vi "HDF5_Write_Filter_Record.vi"(0 "Filter_Refs":T2 {"Filter_Group_ref" format="%.0x"; "TimeStamp_dset" format="%.0x"; "Filter_dset" format="%.0x"}, 5 "Config.FP_User.1.FilterEnab":T1=enum."Step 1", 11 "error in":errorcluster) -> (15 "error out":errorcluster)   [LabVIEW 2018]
doc: "Write a single Noise<x> record with timestamp:\nNoise1\n NoiseInfo - cluster with Timestamp and other metadata for this record\n SummdSpectrum - 1024 element Double array (waveform)"
uses:
  HDF5_Filter_refs.ctl
  <vilib>/addons/h5labview2/base/hid_t.ctl
  Controls/RadioButtons/FilterEnableRadio.ctl
  <vilib>/addons/h5labview2/base/lib_path.vi
  <vilib>/addons/h5labview2/base/H5Equery.vi
  <vilib>/addons/h5labview2/dataset/H5Dwrite.llb/H5Dwrite.xnode
  <vilib>/addons/h5labview2/dataset/H5D.lvlib
  <vilib>/addons/h5labview2/space/H5S.lvlib
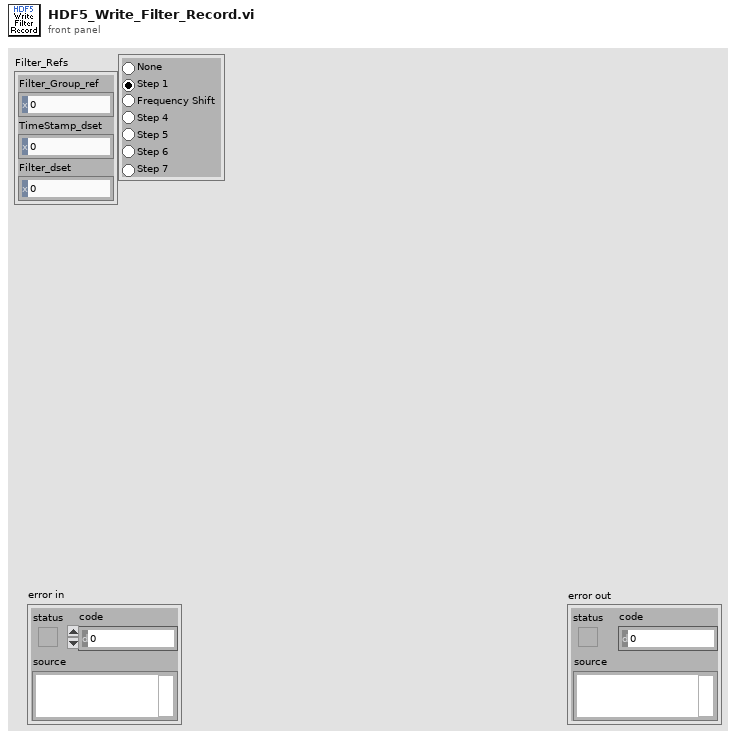
[diagram p1: front panel]
types:
  T1 = typedef "FilterEnableRadio.ctl" = enum32{"None", "Step 1", "Frequency Shift", "Step 4", "Step 5", "Step 6", "Step 7"}
  T2 = typedef "HDF5_Filter_refs.ctl" = cluster{"Filter_Group_ref":T3, "TimeStamp_dset":T3, "Filter_dset":T3}
  T3 = typedef "hid_t.ctl" = i32
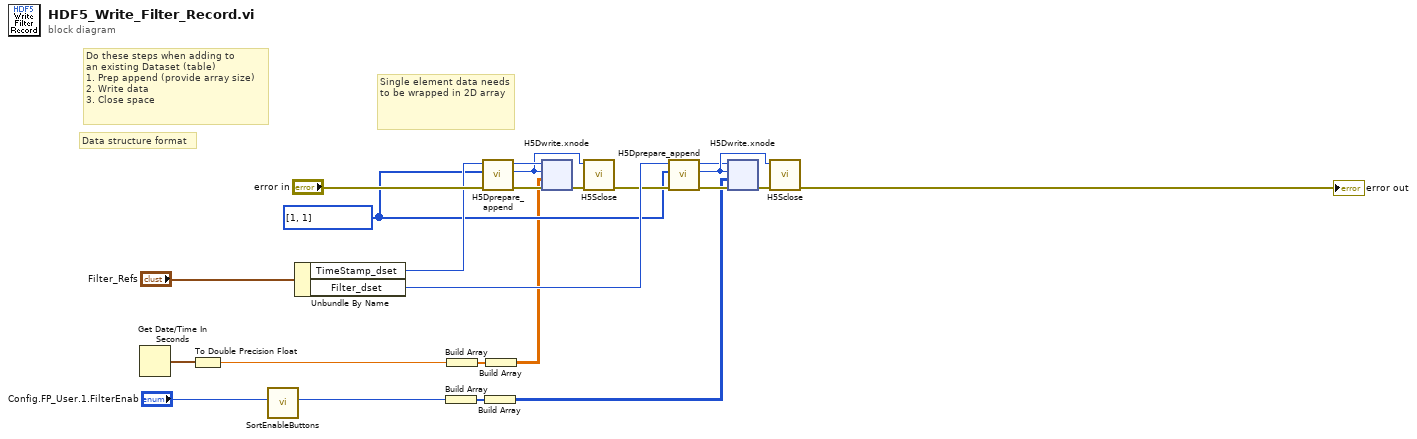
[diagram p0: block diagram]
diagram:
  w7 = u64[] [1, 1] ("append dims")
  # "Single element data needs to be wrapped in 2D array"
  # "Data structure format"
  # "Do these steps when adding to \nan existing Dataset (table)\n1. Prep append (provide array size)\n2. Write data\n3. Close space"
  n1 = Get Date/Time In Seconds() -> (seconds since 1Jan1904=w15:timestamp)
  n2 = To Double Precision Float(number=w15) -> (double precision float=w3:dbl)
  n3 = call "SortEnableButtons.vi"("Radio Buttons"="Config.FP_User.1.FilterEnab") -> ("FilterStage"=w1:u8)  [unwired: 8 in, 2 out]
  n4 = Unbundle By Name("Filter_Refs") -> ("TimeStamp_dset"=w8:T3, "Filter_dset"=w16:T3)
  n5 = Build Array(w1) -> (w19:u8[])
  n6 = Build Array(w3) -> (w6:dbl[])
  n7 = call <vilib>:"H5Dprepare_append.vi"("error in (no error)"="error in", "append dims"=w7, "dset in"=w8) -> ("error out"=w11:errorcluster, "space out"=w13:T3, "dset out"=w14:T3)  [unwired: 5 in, 1 out]
  n8 = Build Array(w19) -> (w18:u8[][])
  n9 = Build Array(w6) -> (w5:dbl[][])
  n10 = xnode "H5Dwrite.xnode"("error in (no error)"=w11, "data"=w5, "file space"=w13, "ref in"=w14) -> ("error out"=w12:errorcluster)  [unwired: 3 in, 2 out]
  n11 = call <vilib>:"H5Sclose.vi"("error in (no error)"=w12, "space in"=w13) -> ("error out"=w10:errorcluster)  [unwired: 9 in]
  n12 = call <vilib>:"H5Dprepare_append.vi"("error in (no error)"=w10, "append dims"=w7, "dset in"=w16) -> ("error out"=w23:errorcluster, "space out"=w21:T3, "dset out"=w20:T3)  [unwired: 5 in, 1 out]
  n13 = xnode "H5Dwrite.xnode"("error in (no error)"=w23, "data"=w18, "file space"=w21, "ref in"=w20) -> ("error out"=w22:errorcluster)  [unwired: 3 in, 2 out]
  n14 = call <vilib>:"H5Sclose.vi"("error in (no error)"=w22, "space in"=w21) -> ("error out"=→"error out":errorcluster)  [unwired: 9 in]
